vi "constructor.vi"(8 "error in (no error)":errorcluster, 11 "singleton in":refnum<class "singleton.lvclass">) -> (0 "error out":errorcluster, 3 "singleton out":refnum<class "singleton.lvclass">)   [LabVIEW 2020, in "singleton.lvclass"]
uses:
  singleton.lvclass
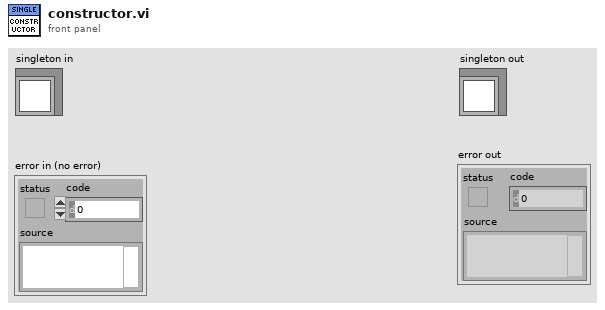
[diagram p1: front panel]
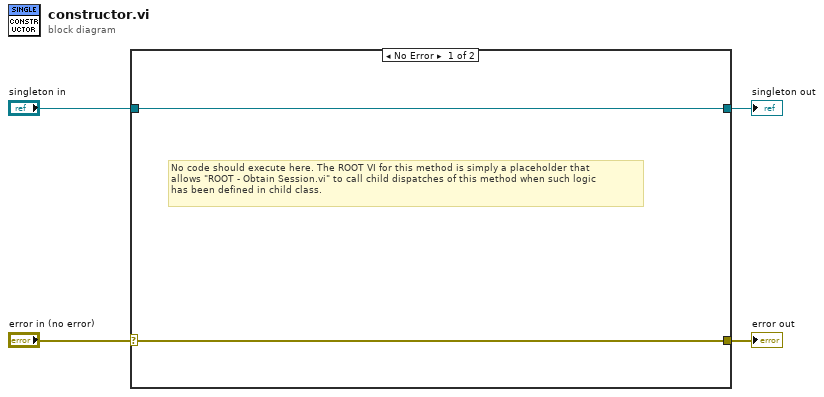
[diagram p0: block diagram]
diagram:
  n1 = case shown="No Error" "error in (no error)" {
    selector: "error in (no error)" -> [w5 w8]
    tunnel: [w5 w8] -> w3
    tunnel: [w6 w7] -> w1
    tunnel: "singleton in" -> [w6 w7]
    frame No Error {
      # "No code should execute here. The ROOT VI for this method is simply a placeholder that\nallows \"ROOT - Obtain Session.vi\" to call child dispatches of this method when such logic\nhas been defined in child class."
    }
    frame Error {
    }
  }
  "error out" <- w3
  "singleton out" <- w1
